vi "Controller Interface Button.vi"() -> ()   [LabVIEW 2023]
uses:
  ButtonCommands.ctl
panel:
  in  "Controller Interface":bool
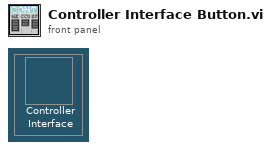
[diagram p1: front panel]
types:
  T1 = typedef "ButtonCommands.ctl" = enum16{"No Command - Error", "Load Buttons", "Remove Buttons", "Get User Event"}
  T2 = enum8{"Enabled", "Disabled", "Disabled and Grayed Out"}
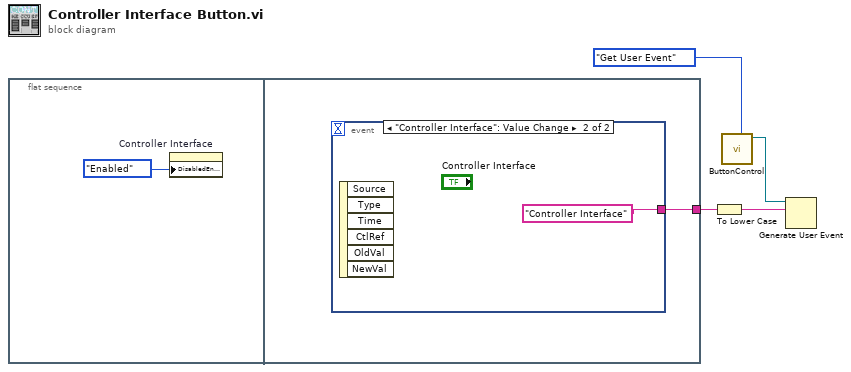
[diagram p0: block diagram]
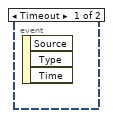
[diagram p2: hidden frame]
diagram:
  n1 = flat-sequence {
    tunnel: [w6] -> w3
    frame #0 {
      n2 = property on="Controller Interface" class="Bool"("DisabledEnum"=T2."Enabled" ("Disabled")) -> ()  [unwired: 2 in, 2 out]
    }
    frame #1 {
      n3 = event shown="[1] \"Controller Interface\": Value Change" {
        selector: _ -> [_ _]
        dyn-events: _ -> [_ _]
        timeout: _ -> [_ _]
        tunnel: [_ "Controller Interface"] -> w6
        event Timeout {
          n4 = event-data() -> ()  [unwired: 1 in, 3 out]
        }
        event "Controller Interface": Value Change {
          n5 = event-data() -> ()  [unwired: 1 in, 6 out]
        }
      }
    }
  }
  n6 = To Lower Case(string=w3) -> (all lower case string=w4:string)
  n7 = call "ButtonControl.vi"("SubPanel Command"=ButtonCommands."Get User Event") -> ("user event Out"=w1:refnum<user-event>)  [unwired: 8 in, 1 out]
  n8 = Generate User Event(user event=w1, event data cluster=w4) -> ()  [unwired: 2 in, 2 out]
